vi "Create All Message Queues.vi"(8 "error in (no error)":errorcluster) -> (0 "error out":errorcluster, 3 "Message Queues out":T1)   [LabVIEW 2019, in "MainController.lvlib"]
doc: "This VI creates and initializes all the message queues for your application. If your application requires more than one message queue, right-click the \"Message Queues\" constant above and select Open Type Def. Add the new Message Queue(s) to the type definition, then initialize them in this VI."
uses:
  MainController.lvlib
  All Message Queues.ctl
  Cluster - MainControllerMessage.ctl
  Enum - MainState.ctl
  AutoMode/Cluster - AutoModeMessage.ctl
  AutoMode/Enum - AutoModeState.ctl
  ManualMode/Cluster - ManualModeMessageCluster.ctl
  ManualMode/Enum - ManualModeMessage.ctl
  Settings/CTL_MessageCluster.ctl
  Settings/CTL_SettingsMessage.ctl
  AutoMode/AutoMode.lvlib
  Settings/Settings.lvlib
  ManualMode/ManualMode.lvlib
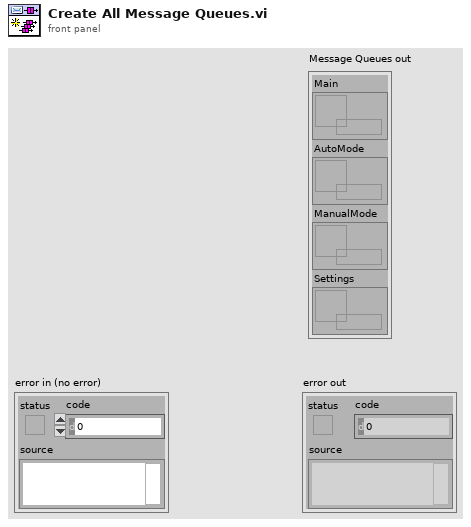
[diagram p1: front panel]
types:
  T1 = typedef "MainController.lvlib/All Message Queues.ctl" = cluster{"Main":refnum<queue>, "AutoMode":refnum<queue>, "ManualMode":refnum<queue>, "Settings":refnum<queue>}
  T2 = typedef "MainController.lvlib/Enum - MainState.ctl" = enum16{"Initialize", "InitUIRefs", "LaunchSettings", "LaunchAutoMode", "LaunchManualMode", "LaunchTestReport", "ConnectHardware", "DisconnectHardware", "HiliteNavItems", "StartAutoMode", "PauseAutoMode", "StopAutoMode", "ShowFlyout", "HideFlyout", "BroadcastSettings", "PickupTestSettings", "BroadcastHW", "AutoTestDone", "DAQStatus", "UpdateCommandBar", "Error", "RecieveError", "Exit"}
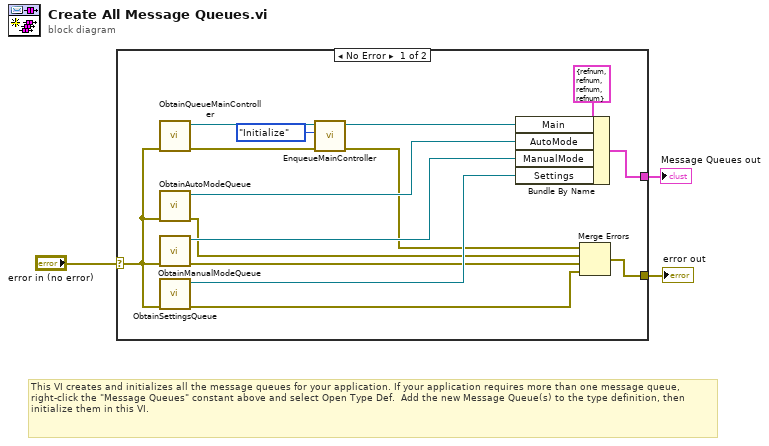
[diagram p0: block diagram]
diagram:
  # "This VI creates and initializes all the message queues for your application. If your application requires more than one message queue, right-click the \"Message Queues\" constant above and select Open Type Def.  Add the new Message Queue(s) to the type definition, then initialize them in this VI."
  n1 = case shown="No Error" "error in (no error)" {
    selector: "error in (no error)" -> [w4 w19]
    tunnel: [w13 w19] -> w3
    tunnel: [w17 _] -> w2
    frame No Error {
      n2 = call "ObtainQueueMainController.vi"("error in (no error)"=w4) -> ("error out"=w16:errorcluster, "MainQueue"=w15:refnum<queue>)  [unwired: 9 in]
      n3 = call "ObtainAutoModeQueue.vi"("error in (no error)"=w4) -> ("error out"=w6:errorcluster, "Queue out"=w8:refnum<queue>)  [unwired: 9 in]
      n4 = call "ObtainManualModeQueue.vi"("error in (no error)"=w4) -> ("error out"=w5:errorcluster, "queue out"=w9:refnum<queue>)  [unwired: 9 in]
      n5 = call "ObtainSettingsQueue.vi"("error in (no error)"=w4) -> ("error out"=w11:errorcluster, "Queue out"=w10:refnum<queue>)  [unwired: 9 in]
      n6 = call "EnqueueMainController.vi"("error in (no error)"=w16, "Message"=Enum_-_MainState."Initialize", "MainQueue"=w15) -> ("error out"=w7:errorcluster, "MainQueue out"=w14:refnum<queue>)  [unwired: 6 in, 1 out]
      n7 = Bundle By Name(cluster=T1 {"Main"=refnum, "AutoMode"=refnum, "ManualMode"=refnum, "Settings"=refnum} ("Message Queues"), "Main"=w14, "AutoMode"=w8, "ManualMode"=w9, "Settings"=w10) -> (w17:T1)
      n8 = Merge Errors(w7, w6, w5, w11) -> (w13:errorcluster)
    }
    frame Error {
    }
  }
  "Message Queues out" <- w2
  "error out" <- w3
